vi "EC60f_InitParam.vi"(8 "error in":errorcluster, 9 "PID Loop Period":dbl=-1.0 format="%#_13g", 10 "Motor Quantity":i32=8, 11 "MotorControl_EC60f":refnum<class "MC_EC60f.lvclass">) -> (0 "error out":errorcluster, 3 "MotorControl_EC60f":refnum<class "MC_EC60f.lvclass">, 4 "EncoderCount":fxp<+,16,16>=1024.0, 6 "PWM (Hz/A)":fxp<+/-,32,16>=13.333328247070312)   [LabVIEW 2015, in "MC_EC60f.lvclass"]
uses:
  MC_EC60f.lvclass
  MotorControl/MotorControl.lvclass
panel:
  in  "MotorConstant(F/V)":dbl=190.0
  in  "PID gain schedule":T1(array[cluster])=[{"PID gains"={"proportional gain (Kc)"=0.001, "integral time (Ti, min)"=100.0, "derivative time (Td, min)"=0.0}, "max value"=100.0}]
  in  "FrictionModel":cluster{"Coeff+":dbl[], "Coeff-":dbl[]}={"Coeff+"=[0.030723, 0.39214], "Coeff-"=[0.037692, 0.34353]}
  out "Motor Quantity dup":i32=8
  in  "TransferRatio":dbl=1.0 format="%#_13g"
  in  "setpoint range (A)":cluster{"output high":dbl, "output low":dbl}={"output high"=0.75, "output low"=-0.25}
  in  "output range (N)":cluster{"setpoint high":dbl, "setpoint low":dbl}={"setpoint high"=150.0, "setpoint low"=3.0}
  in  "Force Rate Limit (N/min)":cluster{"ForceRateLow":dbl, "ForceRateHigh":dbl}={"ForceRateLow"=600.0, "ForceRateHigh"=6000000.0} {"ForceRateHigh" format="%#_13g"; "ForceRateLow" format="%#_13g"}
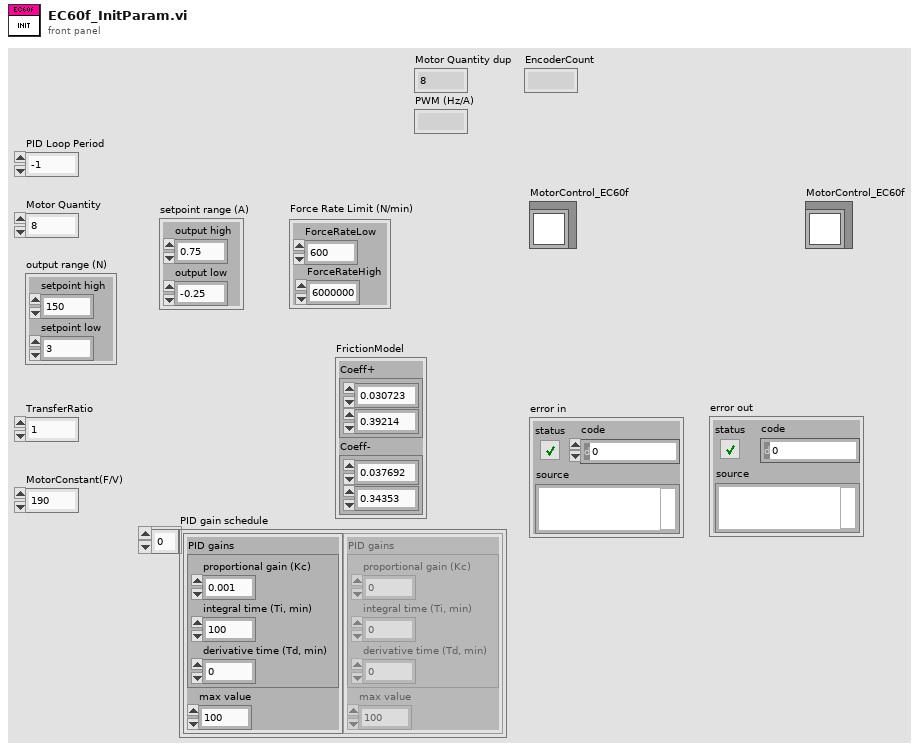
[diagram p1: front panel]
types:
  T1 = cluster{"PID gains":cluster{"proportional gain (Kc)":dbl, "integral time (Ti, min)":dbl, "derivative time (Td, min)":dbl}, "max value":dbl}[]
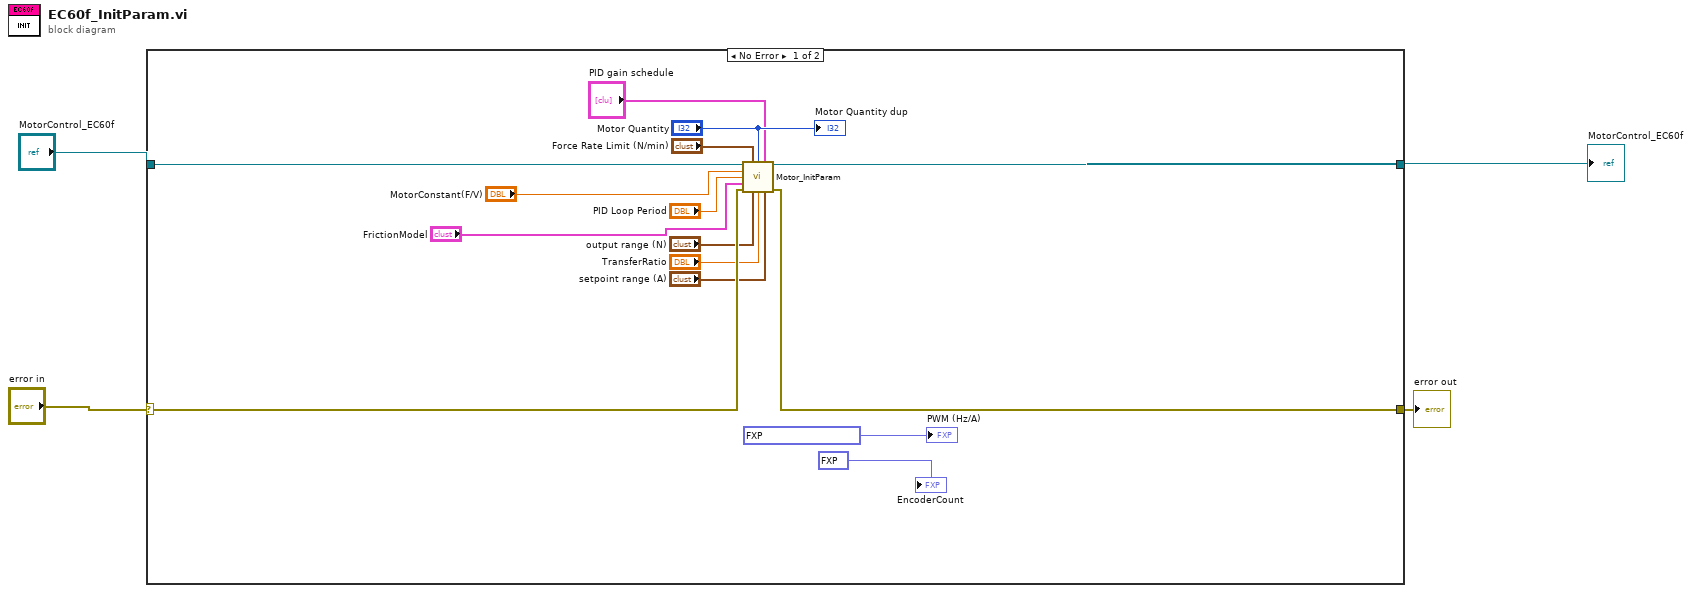
[diagram p0: block diagram]
diagram:
  n1 = case shown="No Error" "error in" {
    selector: "error in" -> [w17 w21]
    tunnel: [w11 w21] -> w1
    tunnel: "MotorControl_EC60f" -> [w19 w20]
    tunnel: [w7 w20] -> w3
    frame No Error {
      n2 = call "Motor_InitParam.vi"("Motor Control In"=w19, "Force Rate Limit (N/min)"="Force Rate Limit (N/min)", "Motor Quantity"="Motor Quantity", "PID gain schedule"="PID gain schedule", "MotorConstant(F/V)"="MotorConstant(F/V)", "PID Loop Period"="PID Loop Period", "FrictionModel"="FrictionModel", "error in (no error)"=w17, "output range (N)"="output range (N)", "TransferRatio"="TransferRatio", "setpoint range (A)"="setpoint range (A)") -> ("Motor Control Out"=w7:refnum<class "MC_EC60f.lvclass">, "error out"=w11:errorcluster)  [unwired: 3 in]
      "Motor Quantity dup" <- "Motor Quantity"
      "PWM (Hz/A)" <- fxp<+/-,32,16> 13.333328247070312 ("PWM (Hz/A) 2")
      "EncoderCount" <- fxp<+,16,16> 1024.0 ("EncoderCount 2")
    }
    frame Error {
    }
  }
  "MotorControl_EC60f" <- w3
  "error out" <- w1
